vi "TEST - LVOOP Is Default Value.vi"(8 "error in (no error)":errorcluster) -> (0 "error out":errorcluster, 2 "Pass":bool)   [LabVIEW 2020, in "test_openg_variant.lvlib"]
uses:
  test_openg_variant.lvlib
  source/library/openg_variant.lvlib
  <vilib>/addons/_JKI Toolkits/Caraya/classes/Test/Test.lvclass
  <vilib>/addons/_JKI Toolkits/Caraya/classes/Assert/Assert.lvclass
  <vilib>/addons/_JKI Toolkits/Caraya/classes/Assert/Assert True.vi
  LVOOP Data/Class 1/Class 1.lvclass
panel:
  out "Test Name":string
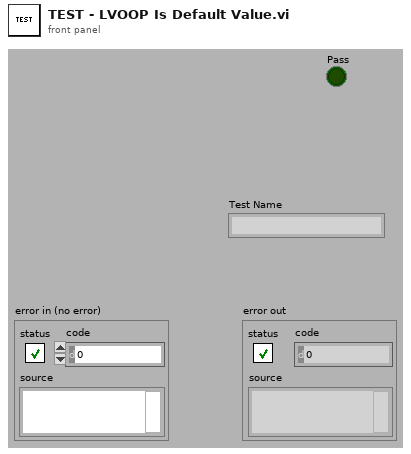
[diagram p1: front panel]
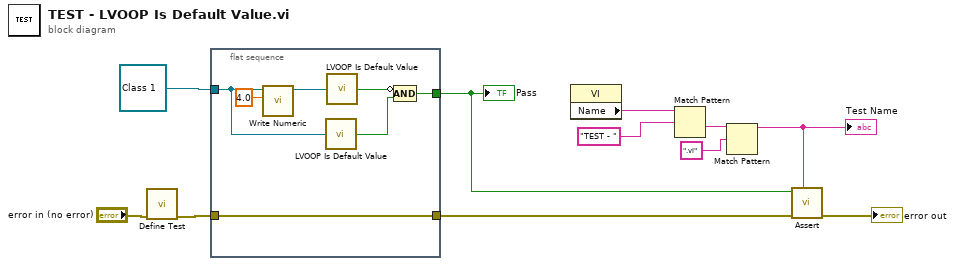
[diagram p0: block diagram]
diagram:
  n1 = call <vilib>:"Define Test.vi"("error in (no error)"="error in (no error)") -> ("error out"=w2:errorcluster)  [unwired: 9 in, 1 out]
  n2 = flat-sequence {
    tunnel: refnum<class "Class 1.lvclass"> refnum ("Class 1 in") -> [w14]
    tunnel: [w13] -> w5
    tunnel: w2 -> [w12]
    tunnel: [w12] -> w1
    frame #0 {
      n3 = call "Write Numeric.vi"("Numeric"=4.0, "Class 1 in"=w14) -> ("Class 1 out"=w16:refnum<class "Class 1.lvclass">)  [unwired: 9 in]
      n4 = call "LVOOP Is Default Value.vi"("Object"=w14) -> ("Is Default Value?"=w15:bool)
      n5 = call "LVOOP Is Default Value.vi"("Object"=w16) -> ("Is Default Value?"=w17:bool)
      n6 = Compound Arithmetic op=AND(invert w17, w15) -> (w13:bool)
    }
  }
  n7 = property class="VI"() -> ("Name"=w9:string)  [unwired: 2 in, 2 out]
  n8 = Match Pattern(string=w9, regular expression="TEST - ") -> (after substring=w10:string)  [unwired: 1 in, 3 out]
  n9 = Match Pattern(string=w10, regular expression=".vi") -> (before substring=w6:string)  [unwired: 1 in, 3 out]
  "Test Name" <- w6
  n10 = call-poly <vilib>:"Assert.vi"("Label"=w6, "error in (no error)"=w1, "True?"=w5) -> ("error out"=→"error out":errorcluster)  [unwired: 7 in, 1 out]
  "Pass" <- w5
